vi "Load_from_Project.vi"(8 "error in (no error)":errorcluster, 9 "index":string, 10 "buildObject":T1, 11 "IB_RegGroup in":refnum<class "IB_RegGroup.lvclass">) -> (0 "error out":errorcluster, 1 "index out":string, 2 "buildObject out":T1, 3 "IB_RegGroup out":refnum<class "IB_RegGroup.lvclass">)   [LabVIEW 2020, in "IB_RegGroup.lvclass"]
uses:
  <vilib>/AppBuilder/IB_Classes/RegGroup/IB_RegGroup.lvclass
  <vilib>/AppBuilder/IB_Classes/RegGroup/IB_RegGroup.lvclass/IB_RegGroup.ctl
  <vilib>/AppBuilder/IB_RW_Project/IB_RW_Project_PropBag_Action.ctl
  <vilib>/AppBuilder/IB_Classes/RegData/IB_RegData.lvclass
  <resource>/Framework/Providers/API/ItemRef.ctl
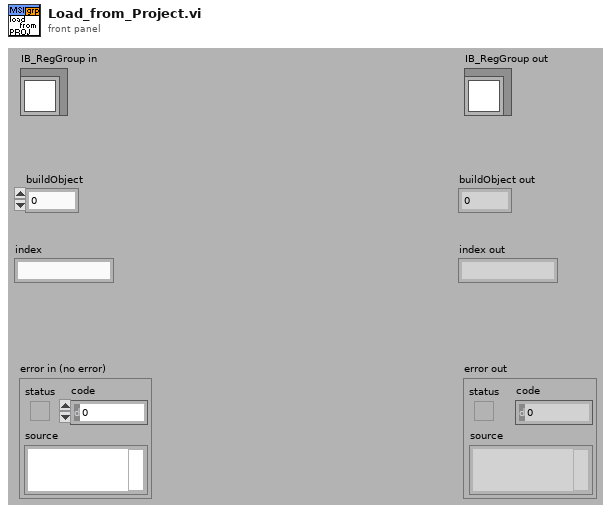
[diagram p1: front panel]
types:
  T1 = typedef "ItemRef.ctl" = u64
  T2 = typedef "IB_RW_Project_PropBag_Action.ctl" = enum16{"read", "write", "clear", "readPrevious", "writePrevious", "clearPrevious"}
  T3 = typedef "IB_RW_Project_RegGroup_Data.ctl" = cluster{"dirTag":string}
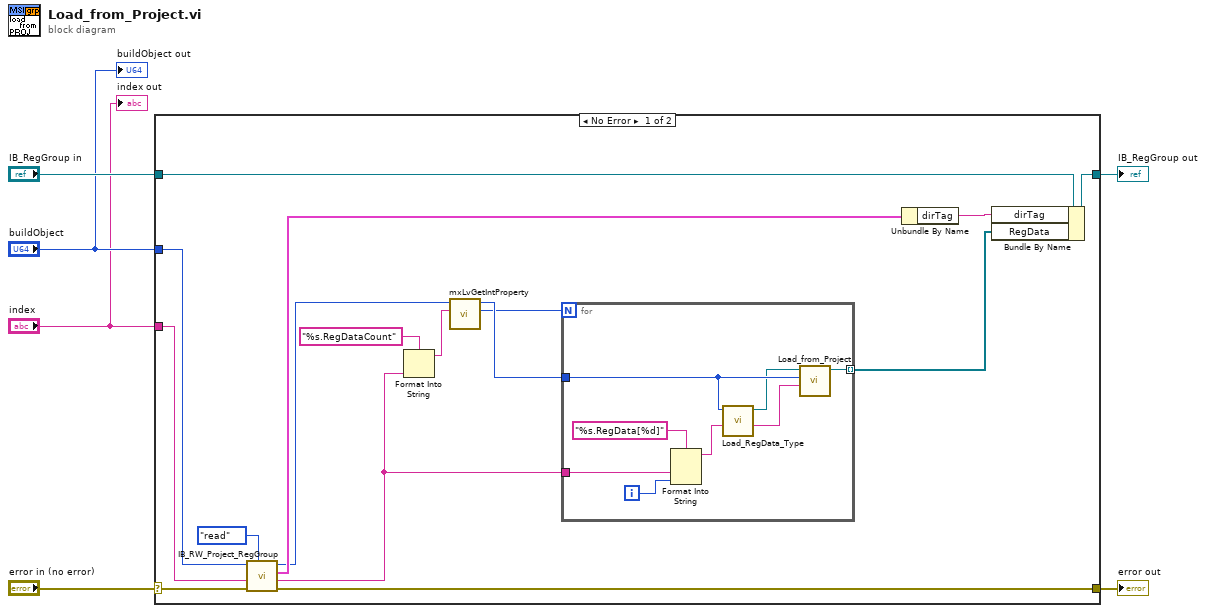
[diagram p0: block diagram]
diagram:
  n1 = case shown="No Error" "error in (no error)" {
    selector: "error in (no error)" -> [w22 w32]
    tunnel: [w21 w32] -> w5
    tunnel: [w15 w31] -> w3
    tunnel: "IB_RegGroup in" -> [w16 w31]
    tunnel: "buildObject" -> [w18 _]
    tunnel: "index" -> [w17 _]
    frame No Error {
      n2 = call <vilib>:"IB_RW_Project_RegGroup.vi"("action"=IB_RW_Project_PropBag_Action."read", "error in (no error)"=w22, "index in"=w17, "buildObject"=w18) -> ("error out"=w21:errorcluster, "index out"=w8:string, "RegGroup"=w19:T3, "buildObject out"=w9:T1)  [unwired: 4 in]
      n3 = Format Into String(format string="%s.RegDataCount", w8) -> (resulting string=w13:string)  [unwired: 2 in, 1 out]
      n4 = call <resource>:"mxLvGetIntProperty.vi"("Tag"=w13, "Item"=w9) -> ("Value"=w10:i32, "Item"=w11:T1)  [unwired: 1 in, 7 out]
      n5 = for {
        N: w10 -> [_]
        tunnel: w11 -> [w24]
        tunnel: w8 -> [w29]
        tunnel: [w27] -> w7 mode=indexing
        i -> [w30]
        n6 = Format Into String(format string="%s.RegData[%d]", w29, w30) -> (resulting string=w26:string)  [unwired: 2 in, 1 out]
        n7 = call <vilib>:"Load_RegData_Type.vi"("index in"=w26, "buildObject"=w24) -> ("index out"=w25:string, "IB_RegData out"=w23:refnum<class "IB_RegData.lvclass">)  [unwired: 7 in, 1 out]
        n8 = call-dynamic "Load_from_Project.vi"("index"=w25, "buildObject"=w24, "IB_RegData in"=w23) -> ("IB_RegData out"=w27:refnum<class "IB_RegData.lvclass">)  [unwired: 5 in, 3 out]
      }
      n9 = Unbundle By Name(w19) -> ("dirTag"=w14:string)
      n10 = Bundle By Name(cluster=w16, "dirTag"=w14, "RegData"=w7) -> (w15:refnum<class "IB_RegGroup.lvclass">)
    }
    frame Error {
    }
  }
  "error out" <- w5
  "IB_RegGroup out" <- w3
  "buildObject out" <- "buildObject"
  "index out" <- "index"
